vi "rate safety.vi"(8 "Max Rate":dbl=1.79e+300, 9 "Cutoff Rate":dbl=0.2, 10 "Desired Rate":dbl, 11 "Encoder Rate":dbl) -> (2 "Output Rate":dbl, 3 "Encoder Rate Out":dbl, 4 "No Rate Read":bool, 6 "Encoder Failure":bool)   [LabVIEW 2014]
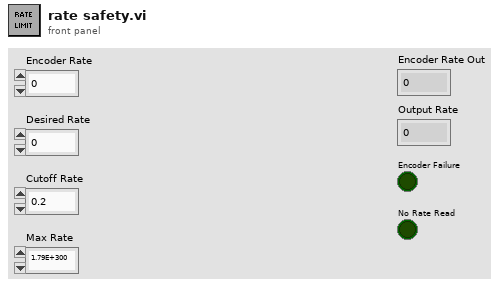
[diagram p1: front panel]
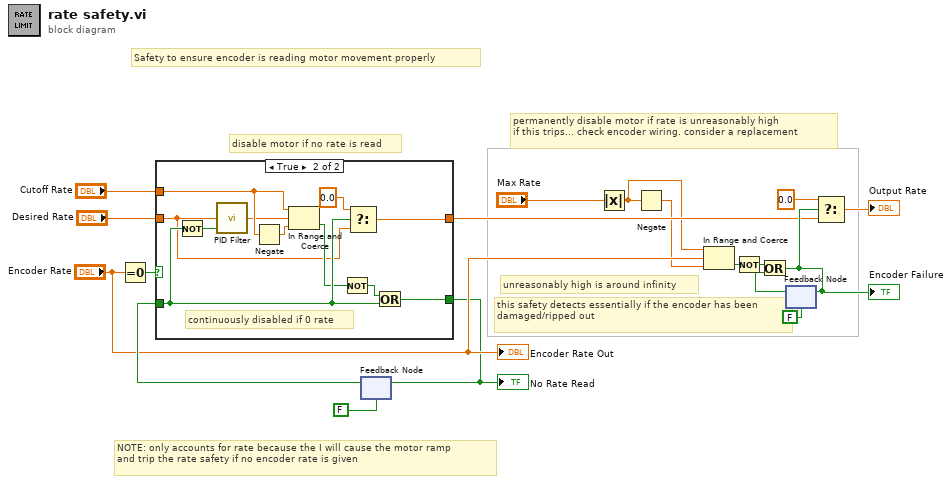
[diagram p0: block diagram]
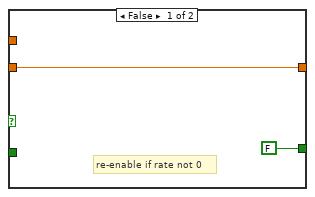
[diagram p2: hidden frame]
diagram:
  # "this safety detects essentially if the encoder has been\ndamaged/ripped out"
  # "unreasonably high is around infinity"
  # "permanently disable motor if rate is unreasonably high\nif this trips... check encoder wiring. consider a replacement"
  # "Safety to ensure encoder is reading motor movement properly"
  # "NOTE: only accounts for rate because the I will cause the motor ramp\nand trip the rate safety if no encoder rate is given"
  # "disable motor if no rate is read"
  n1 = Equal To 0?(x="Encoder Rate") -> (x = 0?=w17:bool)
  n2 = feedback #1(FALSE ("x > y?")) -> (w13:bool)
  n3 = case shown="True" w17 {
    tunnel: "Desired Rate" -> [w20 w21]
    tunnel: [w20 w30] -> w12
    tunnel: [FALSE w28] -> w9
    tunnel: w13 -> [_ w27]
    tunnel: "Cutoff Rate" -> [_ w25]
    frame False {
      # "re-enable if rate not 0"
    }
    frame True {
      # "continuously disabled if 0 rate"
      n4 = Not(x=w27) -> (.not. x?=w24:bool)
      n5 = call "PID Filter.vi"("reinitialize? (F)"=w24, "input"=w21) -> ("output"=w23:dbl)  [unwired: 3 in]
      n6 = Negate(x=w25) -> (-x=w26:dbl)
      n7 = In Range and Coerce(upper limit=w25, x=w23, lower limit=w26) -> (In Range?=w22:bool)  [unwired: 1 out]
      n8 = Not(x=w22) -> (.not. x?=w29:bool)
      n9 = Select(t=0.0, s=w27, f=w21) -> (s? t:f=w30:dbl)
      n10 = Or(x=w29, y=w27) -> (x .or. y?=w28:bool)
    }
  }
  "No Rate Read" <- w9
  n11 = feedback-in #1(w9) -> ()
  n12 = Absolute Value(x="Max Rate") -> (abs(x)=w1:dbl)
  n13 = Negate(x=w1) -> (-x=w3:dbl)
  n14 = In Range and Coerce(upper limit=w1, x="Encoder Rate", lower limit=w3) -> (In Range?=w5:bool)  [unwired: 1 out]
  n15 = Not(x=w5) -> (.not. x?=w4:bool)
  n16 = feedback #2(FALSE ("x > y?")) -> (w6:bool)
  n17 = Or(x=w4, y=w6) -> (x .or. y?=w16:bool)
  "Encoder Failure" <- w16
  n18 = feedback-in #2(w16) -> ()
  n19 = Select(t=0.0, s=w16, f=w12) -> (s? t:f=→"Output Rate":dbl)
  "Encoder Rate Out" <- "Encoder Rate"
